vi "Output Status Query.vi"(8 "error in (no error)":errorcluster, 11 "VISA resource name":refnum<visa-resource-name>) -> (0 "error out":errorcluster, 1 "Standby":bool, 2 "Operating":bool, 3 "VISA resource name out":refnum<visa-resource-name>, 5 "Suspended":bool)   [LabVIEW 2017, in "ADCMT 6240.lvlib"]
doc: "Read output status of the instrument."
uses:
  ADCMT 6240.lvlib
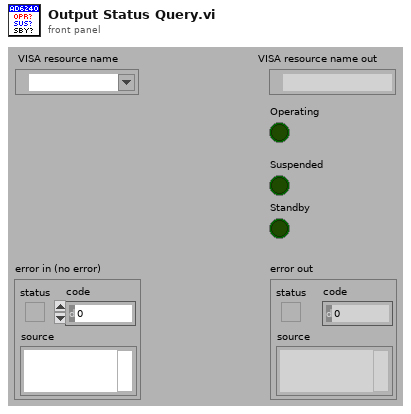
[diagram p1: front panel]
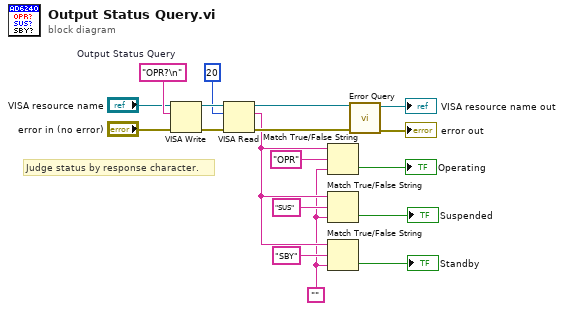
[diagram p0: block diagram]
diagram:
  w1 = ""
  w13 = "OPR?\n"  # Output Status Query
  # "Judge status by response character."
  n1 = VISA Write(VISA resource name="VISA resource name", write buffer=w13, error in (no error)="error in (no error)") -> (VISA resource name out=w18:refnum<visa-resource-name>, error out=w17:errorcluster)  [unwired: 1 out]
  n2 = VISA Read(VISA resource name=w18, byte count=u32 20 ("byte count (20)"), error in (no error)=w17) -> (VISA resource name out=w11:refnum<visa-resource-name>, read buffer=w2:string, error out=w12:errorcluster)  [unwired: 1 out]
  n3 = Match True/False String(2:w1, 3:"OPR", 4:w2) -> (0:→"Operating":bool)  [unwired: 1 out]
  n4 = Match True/False String(2:w1, 3:"SUS", 4:w2) -> (0:→"Suspended":bool)  [unwired: 1 out]
  n5 = Match True/False String(2:w1, 3:"SBY", 4:w2) -> (0:→"Standby":bool)  [unwired: 1 out]
  n6 = call "Error Query.vi"("error in (no error)"=w12, "VISA resource name"=w11) -> ("error out"=→"error out":errorcluster, "VISA resource name out"=→"VISA resource name out":refnum<visa-resource-name>)  [unwired: 6 in, 2 out]
